vi "Keithley 2400 - CurrSource.vi"(8 "Tensão limite:":dbl=31.0, 10 "Corrente aplicada:":dbl=2e-06, 11 "Porta:":refnum<visa-resource-name>="COM5") -> (0 "Corrente:":dbl, 3 "Tensão:":dbl)   [LabVIEW 2011]
uses:
  <vilib>/Instr/_visa.llb/VISA Configure Serial Port (Instr).vi
panel:
  out "error out":errorcluster
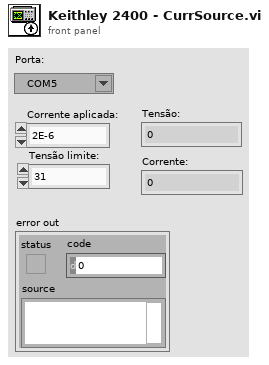
[diagram p1: front panel]
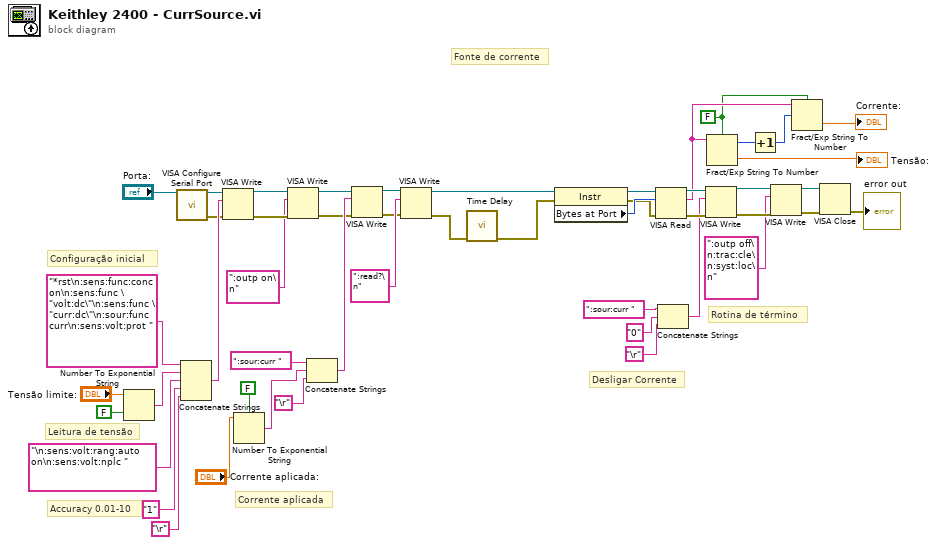
[diagram p0: block diagram]
diagram:
  w7 = FALSE ("use system decimal point (T)")
  # "Rotina de término"
  # "Leitura de tensão"
  # "Configuração inicial"
  # "Desligar Corrente"
  # "Corrente aplicada"
  # "Accuracy 0.01-10"
  # "Fonte de corrente"
  n1 = Number To Exponential String(number="Tensão limite:", 1:FALSE ("use system decimal point (T)")) -> (E-format string=w1:string)  [unwired: 2 in]
  n2 = call-poly "VISA Configure Serial Port"("VISA resource name"="Porta:") -> ("VISA resource name out"=w13:refnum<visa-resource-name>, "error out"=w14:errorcluster)  [unwired: 13 in]
  n3 = Concatenate Strings("*rst\n:sens:func:conc on\n:sens:func \"volt:dc\"\n:sens:func \"curr:dc\"\n:sour:func curr\n:sens:volt:prot " ("string"), w1, "\n:sens:volt:rang:auto on\n:sens:volt:nplc " ("string"), "1" ("string"), "\r") -> (w46:string)
  n4 = VISA Write(VISA resource name=w13, write buffer=w46, error in (no error)=w14) -> (VISA resource name out=w45:refnum<visa-resource-name>, error out=w44:errorcluster)  [unwired: 1 out]
  n5 = Number To Exponential String(number="Corrente aplicada:", 1:FALSE ("use system decimal point (T)")) -> (E-format string=w6:string)  [unwired: 2 in]
  n6 = VISA Write(VISA resource name=w45, write buffer=":outp on\n", error in (no error)=w44) -> (VISA resource name out=w40:refnum<visa-resource-name>, error out=w39:errorcluster)  [unwired: 1 out]
  n7 = Concatenate Strings(":sour:curr " ("string"), w6, "\r") -> (w41:string)
  n8 = VISA Write(VISA resource name=w40, write buffer=w41, error in (no error)=w39) -> (VISA resource name out=w35:refnum<visa-resource-name>, error out=w36:errorcluster)  [unwired: 1 out]
  n9 = VISA Write(VISA resource name=w35, write buffer=":read?\n", error in (no error)=w36) -> (VISA resource name out=w33:refnum<visa-resource-name>, error out=w37:errorcluster)  [unwired: 1 out]
  n10 = call "Time Delay"("error in (no error)"=w37) -> ("error out"=w34:errorcluster)  [unwired: 10 in]
  n11 = property class="Instr"(reference=w33, error in=w34) -> (reference out=w31:refnum<visa-resource-name>, error out=w30:errorcluster, "Bytes at Port"=w32:u32)
  n12 = VISA Read(VISA resource name=w31, byte count=w32, error in (no error)=w30) -> (VISA resource name out=w29:refnum<visa-resource-name>, read buffer=w12:string, error out=w28:errorcluster)  [unwired: 1 out]
  n13 = Concatenate Strings(":sour:curr " ("write buffer"), "0" ("string"), "\r") -> (w25:string)
  n14 = VISA Write(VISA resource name=w29, write buffer=w25, error in (no error)=w28) -> (VISA resource name out=w24:refnum<visa-resource-name>, error out=w23:errorcluster)  [unwired: 1 out]
  n15 = Fract/Exp String To Number(use system decimal point (T)=w7, string=w12) -> (offset past number=w11:i32, number=→"Tensão:":dbl)  [unwired: 2 in]
  n16 = Increment(x=w11) -> (x+1=w10:i32)
  n17 = VISA Write(VISA resource name=w24, write buffer=":outp off\n:trac:cle\n:syst:loc\n", error in (no error)=w23) -> (VISA resource name out=w17:refnum<visa-resource-name>, error out=w16:errorcluster)  [unwired: 1 out]
  n18 = Fract/Exp String To Number(use system decimal point (T)=w7, string=w12, offset=w10) -> (number=→"Corrente:":dbl)  [unwired: 1 in, 1 out]
  n19 = VISA Close(VISA resource name=w17, error in (no error)=w16) -> (error out=→"error out":errorcluster)
